vi "robot.vi"() -> ()   [LabVIEW 2010]
uses:
  <vilib>/robotics/Kinematics/Link/Joint Type.ctl
  <vilib>/robotics/Kinematics/Link/NI_Robotics_Link.lvclass
  <vilib>/robotics/Kinematics/Robot/NI_Robotics_Serial Robot Arm.lvclass
  <vilib>/robotics/Kinematics/Plotting/NI_Robotics_3DKinematics.lvlib
panel:
  out "16bit integer 4":i16
  out "16bit integer 3":i16
  out "16bit integer 2":i16
  out "16bit integer":i16
  in  "Control":dbl[](array[slide]) scale=-90.0..90.0
  in  "stop":bool
  out "3D Picture Control":refnum<vi>(3d-picture)
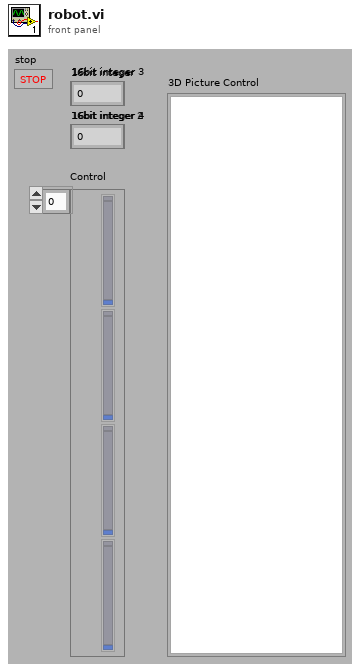
[diagram p1: front panel]
types:
  T1 = typedef "NI_Robotics_Link.lvclass/Joint Type.ctl" = enum16{"Revolute", "Prismatic"}
  T2 = cluster{"twist angle":dbl, "length":dbl, "rotation angle":dbl, "offset distance":dbl, "joint type":T1, "joint coordinate offset":dbl}
  T3 = cluster{"Control[0]":dbl, "Control[1]":dbl, "Control[2]":dbl, "Control[3]":dbl, "Control[4]":dbl, "Control[5]":dbl, "Control[6]":dbl, "Control[7]":dbl, "Control[8]":dbl}
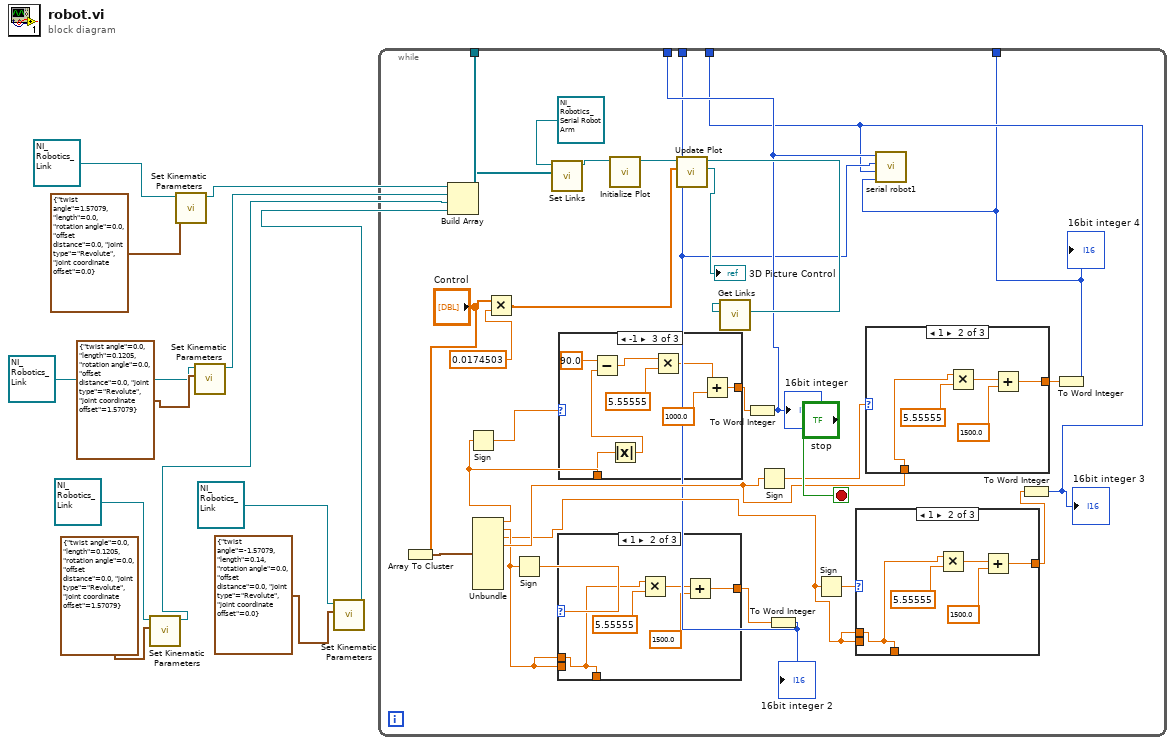
[diagram p0: block diagram]
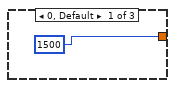
[diagram p2: hidden frame]
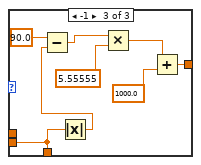
[diagram p3: hidden frame]
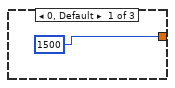
[diagram p4: hidden frame]
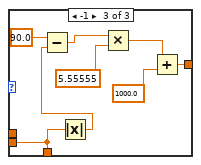
[diagram p5: hidden frame]
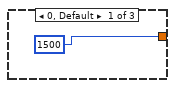
[diagram p6: hidden frame]
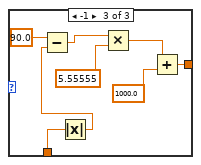
[diagram p7: hidden frame]
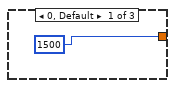
[diagram p8: hidden frame]
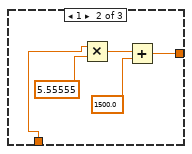
[diagram p9: hidden frame]
diagram:
  n1 = call <vilib>:"Set Kinematic Parameters.vi"("kinematic parameters"=T2 {"twist angle"=0.0, "length"=0.1205, "rotation angle"=0.0, "offset distance"=0.0, "joint type"=enum."Revolute", "joint coordinate offset"=1.57079}, "link in"=refnum<class "NI_Robotics_Link.lvclass"> refnum) -> ("link out"=w2:refnum<class "NI_Robotics_Link.lvclass">)  [unwired: 8 in, 1 out]
  n2 = call <vilib>:"Set Kinematic Parameters.vi"("kinematic parameters"=T2 {"twist angle"=1.57079, "length"=0.0, "rotation angle"=0.0, "offset distance"=0.0, "joint type"=enum."Revolute", "joint coordinate offset"=0.0}, "link in"=refnum<class "NI_Robotics_Link.lvclass"> refnum) -> ("link out"=w11:refnum<class "NI_Robotics_Link.lvclass">)  [unwired: 8 in, 1 out]
  n3 = call <vilib>:"Set Kinematic Parameters.vi"("kinematic parameters"=T2 {"twist angle"=0.0, "length"=0.1205, "rotation angle"=0.0, "offset distance"=0.0, "joint type"=enum."Revolute", "joint coordinate offset"=1.57079}, "link in"=refnum<class "NI_Robotics_Link.lvclass"> refnum) -> ("link out"=w7:refnum<class "NI_Robotics_Link.lvclass">)  [unwired: 8 in, 1 out]
  n4 = call <vilib>:"Set Kinematic Parameters.vi"("kinematic parameters"=T2 {"twist angle"=-1.57079, "length"=0.14, "rotation angle"=0.0, "offset distance"=0.0, "joint type"=enum."Revolute", "joint coordinate offset"=0.0}, "link in"=refnum<class "NI_Robotics_Link.lvclass"> refnum) -> ("link out"=w1:refnum<class "NI_Robotics_Link.lvclass">)  [unwired: 8 in, 1 out]
  n5 = Build Array(w11, w7, w2, w1) -> (w10:refnum<class "NI_Robotics_Link.lvclass">[])
  n6 = while {
    tunnel: w10 -> [w40]
    tunnel: [w17] -> _
    tunnel: [w16] -> _
    tunnel: [w15] -> _
    tunnel: [w14] -> _
    stop <- "stop" stop-if-true
    n7 = Array To Cluster(array="Control") -> (cluster=w30:T3)
    n8 = Unbundle(w30) -> ("Control[0]"=w28:dbl, "Control[1]"=w19:dbl, "Control[2]"=w18:dbl, "Control[3]"=w21:dbl)  [unwired: 5 out]
    n9 = Sign(1:w28) -> (0:w29:dbl)
    n10 = Multiply(x="Control", y=0.0174503) -> (x*y=w33:dbl[])
    n11 = Sign(1:w19) -> (0:w26:dbl)
    n12 = call <vilib>:"Set Links.vi"("links"=w40, "serial arm in"=refnum<class "NI_Robotics_Serial Robot Arm.lvclass"> refnum) -> ("serial arm out"=w38:refnum<class "NI_Robotics_Serial Robot Arm.lvclass">)  [unwired: 8 in, 1 out]
    n13 = case shown="1" w26 {
      tunnel: [_ w42 w47] -> _
      tunnel: [1500 w43 w48] -> w25
      tunnel: w19 -> [_ _ w47]
      tunnel: w19 -> [_ w42 _]
      frame 0, Default {
      }
      frame 1 {
        n14 = Multiply(x=w42, y=5.55555) -> (x*y=w45:dbl)
        n15 = Add(x=w45, y=1500.0) -> (x+y=w43:dbl)
      }
      frame -1 {
        n16 = Absolute Value(x=w47) -> (abs(x)=w52:dbl)
        n17 = Subtract(x=90.0, y=w52) -> (x-y=w49:dbl)
        n18 = Multiply(x=w49, y=5.55555) -> (x*y=w54:dbl)
        n19 = Add(x=w54, y=1000.0) -> (x+y=w48:dbl)
      }
    }
    n20 = case shown="-1" w29 {
      tunnel: w28 -> [_ w84 w94]
      tunnel: [1500 w85 w89] -> w27
      frame 0, Default {
      }
      frame 1 {
        n21 = Multiply(x=w84, y=5.55555) -> (x*y=w87:dbl)
        n22 = Add(x=w87, y=1500.0) -> (x+y=w85:dbl)
      }
      frame -1 {
        n23 = Absolute Value(x=w94) -> (abs(x)=w93:dbl)
        n24 = Subtract(x=90.0, y=w93) -> (x-y=w90:dbl)
        n25 = Multiply(x=w90, y=5.55555) -> (x*y=w96:dbl)
        n26 = Add(x=w96, y=1000.0) -> (x+y=w89:dbl)
      }
    }
    n27 = call <vilib>:"Initialize Plot.vi"("serial arm in"=w38) -> ("serial arm out"=w35:refnum<class "NI_Robotics_Serial Robot Arm.lvclass">)  [unwired: 9 in, 1 out]
    n28 = call <vilib>:"Update Plot.vi"("joint positions"=w33, "serial arm in"=w35) -> ("serial arm scene"=→"3D Picture Control":refnum<vi>, "serial arm out"=w36:refnum<class "NI_Robotics_Serial Robot Arm.lvclass">)  [unwired: 7 in, 1 out]
    n29 = call <vilib>:"Get Links.vi"("serial arm in"=w36) -> ()  [unwired: 8 in, 3 out]
    n30 = To Word Integer(number=w27) -> (16bit integer=w17:i16)
    "16bit integer" <- w17
    n31 = Sign(1:w21) -> (0:w22:dbl)
    n32 = To Word Integer(number=w25) -> (16bit integer=w16:i16)
    "16bit integer 2" <- w16
    n33 = Sign(1:w18) -> (0:w24:dbl)
    n34 = case shown="1" w24 {
      tunnel: [_ w56 w61] -> _
      tunnel: [1500 w57 w62] -> w23
      tunnel: w18 -> [_ _ w61]
      tunnel: w18 -> [_ w56 _]
      frame 0, Default {
      }
      frame 1 {
        n35 = Multiply(x=w56, y=5.55555) -> (x*y=w59:dbl)
        n36 = Add(x=w59, y=1500.0) -> (x+y=w57:dbl)
      }
      frame -1 {
        n37 = Absolute Value(x=w61) -> (abs(x)=w66:dbl)
        n38 = Subtract(x=90.0, y=w66) -> (x-y=w63:dbl)
        n39 = Multiply(x=w63, y=5.55555) -> (x*y=w68:dbl)
        n40 = Add(x=w68, y=1000.0) -> (x+y=w62:dbl)
      }
    }
    n41 = case shown="1" w22 {
      tunnel: w21 -> [_ w70 w80]
      tunnel: [1500 w71 w75] -> w20
      frame 0, Default {
      }
      frame 1 {
        n42 = Multiply(x=w70, y=5.55555) -> (x*y=w73:dbl)
        n43 = Add(x=w73, y=1500.0) -> (x+y=w71:dbl)
      }
      frame -1 {
        n44 = Absolute Value(x=w80) -> (abs(x)=w79:dbl)
        n45 = Subtract(x=90.0, y=w79) -> (x-y=w76:dbl)
        n46 = Multiply(x=w76, y=5.55555) -> (x*y=w82:dbl)
        n47 = Add(x=w82, y=1000.0) -> (x+y=w75:dbl)
      }
    }
    n48 = To Word Integer(number=w23) -> (16bit integer=w15:i16)
    "16bit integer 3" <- w15
    n49 = To Word Integer(number=w20) -> (16bit integer=w14:i16)
    "16bit integer 4" <- w14
    n50 = call "serial robot1.vi"("Numeric"=w17, "Numeric 2"=w16, "Numeric 3"=w15, "Numeric 4"=w14) -> ()  [unwired: 7 in]
  }
